vi "API_GET.vi"(6 "error in (no error)":errorcluster, 8 "endpoint":string, 9 "DB_API.lvclass":refnum<class "DB_API.lvclass">) -> (0 "error out":errorcluster, 2 "body":string, 3 "output cluster":refnum<class "DB_API.lvclass">)   [LabVIEW 2024, in "DB_API.lvclass"]
uses:
  DB_API.lvclass
  DB_API.lvclass/DB_API.ctl
  <vilib>/httpClient/LabVIEWHTTPClient.lvlib
panel:
  out "concatenated string":string
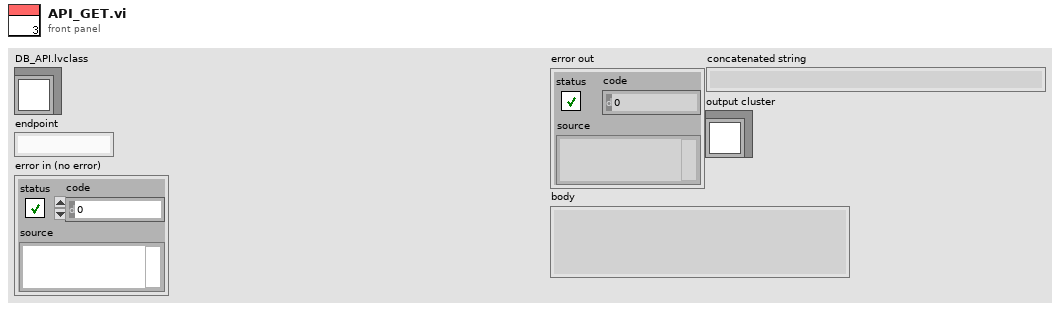
[diagram p1: front panel]
types:
  T1 = typedef "LabVIEWHTTPClient.lvlib/ClientHandle.ctl" = refnum<k1>
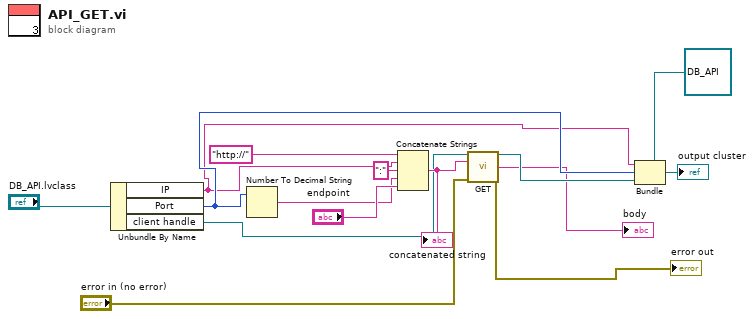
[diagram p0: block diagram]
diagram:
  n1 = Unbundle By Name("DB_API.lvclass") -> ("IP"=w5:string, "Port"=w9:u32, "client handle"=w12:T1)
  n2 = Number To Decimal String(number=w9) -> (decimal integer string=w2:string)  [unwired: 1 in]
  n3 = Concatenate Strings("http://" ("string"), w5, ":" ("string"), w2, "endpoint") -> (w13:string)
  "concatenated string" <- w13
  n4 = call <vilib>:"GET.vi"("client handle"=w12, "url"=w13, "error in (no error)"="error in (no error)") -> ("client handle out"=w8:T1, "body"=→"body":string, "error out"=→"error out":errorcluster)  [unwired: 9 in, 1 out]
  n5 = Bundle(cluster=refnum<class "DB_API.lvclass"> refnum ("DB_API.lvclass"), w5, w9, w8) -> (→"output cluster":refnum<class "DB_API.lvclass">)
